vi "Display.vi"(8 "error in (no error)":errorcluster, 10 "SubPnl Refnum":refnum<vi>, 11 "Slide in":refnum<class "Slide.lvclass">) -> (0 "error out":errorcluster, 3 "Slide out":refnum<class "Slide.lvclass">)   [LabVIEW 2017, in "Slide.lvclass"]
uses:
  Slide.lvclass
  Slide.lvclass/Slide.ctl
panel:
  out "2D Picture":picture
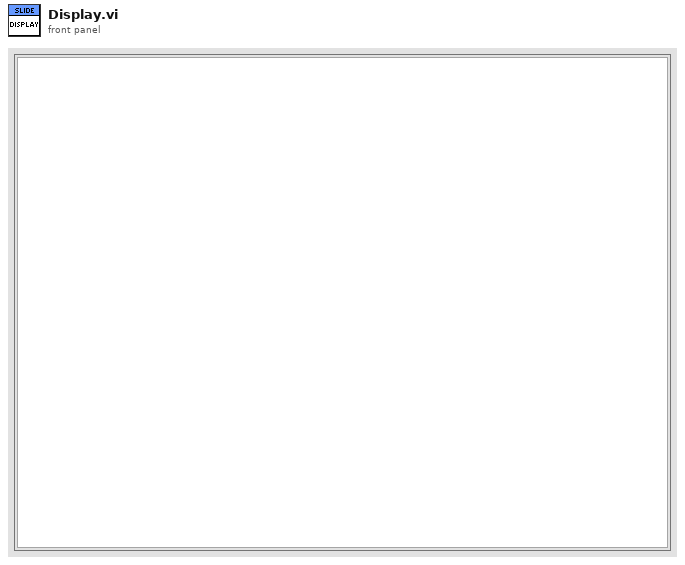
[diagram p1: front panel]
types:
  T1 = typedef "Slide.lvclass/SlideType.ctl" = enum16{"Image", "FP", "BD", "VI-Run"}
  T2 = typedef "imagedata.ctl" = cluster{"image type":i32, "image depth":i32, "image":u8[], "mask":u8[], "colors":u32[], "Rectangle":cluster{"left":i16, "top":i16, "right":i16, "bottom":i16}}
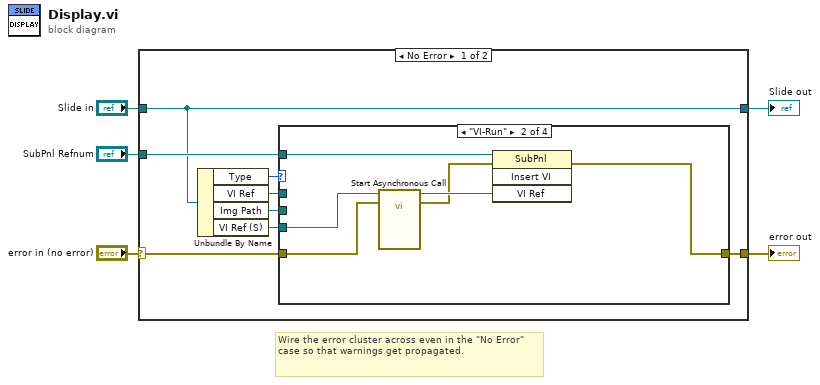
[diagram p0: block diagram]
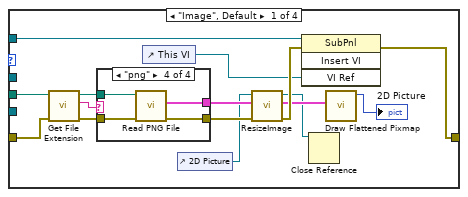
[diagram p2: hidden frame]
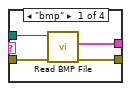
[diagram p3: hidden frame]
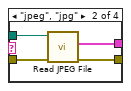
[diagram p4: hidden frame]
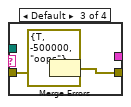
[diagram p5: hidden frame]
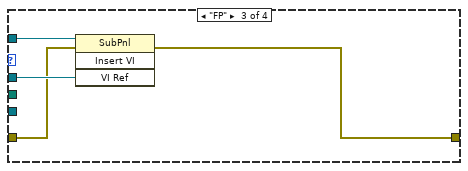
[diagram p6: hidden frame]
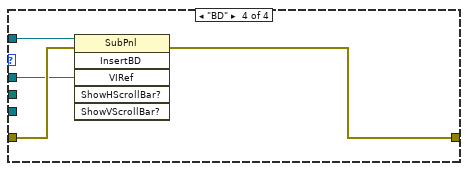
[diagram p7: hidden frame]
diagram:
  # "Wire the error cluster across even in the \"No Error\"\ncase so that warnings get propagated."
  n1 = case shown="No Error" "error in (no error)" {
    selector: "error in (no error)" -> [w13 w59]
    tunnel: [w8 w59] -> w4
    tunnel: [w11 w58] -> w2
    tunnel: "Slide in" -> [w11 w58]
    tunnel: "SubPnl Refnum" -> [w12 _]
    frame No Error {
      n2 = Unbundle By Name(w11) -> ("Type"=w10:T1, "VI Ref"=w9:refnum<vi>, "Img Path"=w7:path, "VI Ref (S)"=w6:refnum<vi>)
      n3 = case shown="\"VI-Run\"" w10 {
        tunnel: w12 -> [w20 w49 w53 w57]
        tunnel: w9 -> [_ _ w52 w54]
        tunnel: w13 -> [w26 w45 w51 w56]
        tunnel: [w19 w48 w50 w55] -> w8
        tunnel: w7 -> [w27 _ _ _]
        tunnel: w6 -> [_ w47 _ _]
        frame "Image", Default {
          n4 = call <vilib>:"Get File Extension.vi"("error in (no error)"=w26, "file"=w27) -> ("error out"=w21:errorcluster, "lowercase file extension"=w23:string, "dup file"=w22:path)  [unwired: 5 in, 2 out]
          n5 = case shown="\"png\"" w23 {
            tunnel: [w30 w33 _ w43] -> w25
            tunnel: w22 -> [w32 w35 _ w42]
            tunnel: w21 -> [w31 w36 w39 w41]
            tunnel: [w29 w34 w38 w40] -> w16
            frame "bmp" {
              n6 = call <vilib>:"Read BMP File.vi"("error in (no error)"=w31, "path to BMP file"=w32) -> ("error out"=w29:errorcluster, "image data"=w30:T2)  [unwired: 7 in, 1 out]
            }
            frame "jpeg", "jpg" {
              n7 = call <vilib>:"Read JPEG File.vi"("error in (no error)"=w36, "path to JPEG file"=w35) -> ("error out"=w34:errorcluster, "image data"=w33:T2)  [unwired: 7 in, 1 out]
            }
            frame Default {
              n8 = Merge Errors(errorcluster {"status"=TRUE, "code"=-500000, "source"="oops"} ("error constant"), w39) -> (w38:errorcluster)
            }
            frame "png" {
              n9 = call <vilib>:"Read PNG File.vi"("error in (no error)"=w41, "path to PNG file"=w42) -> ("error out"=w40:errorcluster, "image data"=w43:T2)  [unwired: 7 in, 1 out]
            }
          }
          n10 = control-ref of="This VI"() -> (w18:refnum<vi>)
          n11 = control-ref of="2D Picture"() -> (w15:refnum<vi>)
          n12 = call "ResizeImage.vi"("error in (no error)"=w16, "Image Data"=w25, "2D Picture Ref"=w15) -> ("error out"=w28:errorcluster, "Image Data (dup)"=w17:T2, "Zoomed Picture Ref"=w14:refnum<vi>)  [unwired: 6 in]
          n13 = invoke class="SubPnl" method="Insert VI"(reference=w20, error in=w28, "VI Ref"=w18) -> (error out=w19:errorcluster)  [unwired: 1 in, 3 out]
          n14 = Close Reference(reference=w14) -> ()  [unwired: 1 in, 1 out]
          n15 = call <vilib>:"Draw Flattened Pixmap.vi"("image data"=w17) -> ("new picture"=→"2D Picture":picture)  [unwired: 8 in]
        }
        frame "VI-Run" {
          n16 = call-by-ref "Start Asynchronous Call"(reference=w47, error in=w45) -> (reference out=w46:refnum<vi>, error out=w44:errorcluster)  [unwired: 12 in]
          n17 = invoke class="SubPnl" method="Insert VI"(reference=w49, error in=w44, "VI Ref"=w46) -> (error out=w48:errorcluster)  [unwired: 1 in, 3 out]
        }
        frame "FP" {
          n18 = invoke class="SubPnl" method="Insert VI"(reference=w53, error in=w51, "VI Ref"=w52) -> (error out=w50:errorcluster)  [unwired: 1 in, 3 out]
        }
        frame "BD" {
          n19 = invoke class="SubPnl" method="InsertBD"(reference=w57, error in=w56, "VIRef"=w54) -> (error out=w55:errorcluster)  [unwired: 3 in, 5 out]
        }
      }
    }
    frame Error {
    }
  }
  "error out" <- w4
  "Slide out" <- w2
